vi "shift registers.vi"() -> ()   [LabVIEW 2022 SP3]
panel:
  out "Previous iteration":dbl
  out "Top Iteration":dbl
  out "Output":dbl
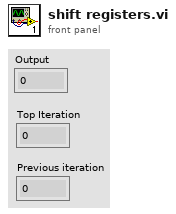
[diagram p1: front panel]
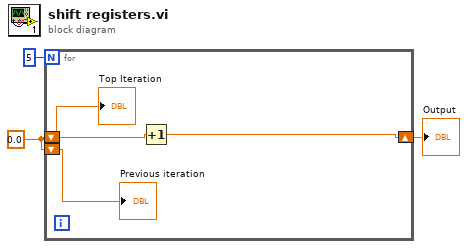
[diagram p0: block diagram]
diagram:
  w1 = 0.0
  n1 = for {
    N: 5 -> [_]
    shift-right: [w6] -> w2
    shift-left: w1 -> [w5]
    shift-left: w1 -> [w4]
    n2 = Increment(x=w5) -> (x+1=w6:dbl)
    "Top Iteration" <- w5
    "Previous iteration" <- w4
  }
  "Output" <- w2
